vi "Radau5_Initialization of Implicit RK Data.vi"(3 "Simulation Data":T5 {"Absolute tolerance" format="%.1e"; "Relative tolerance" format="%.1e"; "Output of T" format="%.1e"; "proposed step size" format="%.1e"; "min step size" format="%.1e"; "max step size" format="%.1e"; "final time" format="%.1e"; "step size" format="%.1e"; "initial time" format="%.1e"}) -> (1 "Implicit RK Data":T1)   [LabVIEW 2020, in "NI_DAE.lvlib"]
uses:
  <vilib>/gmath/NI_DAE.lvlib
  <vilib>/gmath/dae.llb/Radau5_Simulation Data.ctl
  <vilib>/gmath/dae.llb/Radau5_Diag Eval Stage.ctl
  <vilib>/gmath/dae.llb/Radau5_Implicit RK Data.ctl
  <vilib>/gmath/dae.llb/Radau5_RK Status.ctl
  <vilib>/Analysis/Matrix/Datatypes/RealMatrix.ctl
  <vilib>/Analysis/Matrix/Datatypes/ComplexMatrix.ctl
  <vilib>/Analysis/Matrix/Numeric/Conversions/Array To Matrix - CA2.vi
  <vilib>/Analysis/Matrix/Numeric/Conversions/Array To Matrix - RA2.vi
  <vilib>/Analysis/Matrix/NI_Matrix.lvlib
panel:
  in  "Implicit RK Data Type":T1
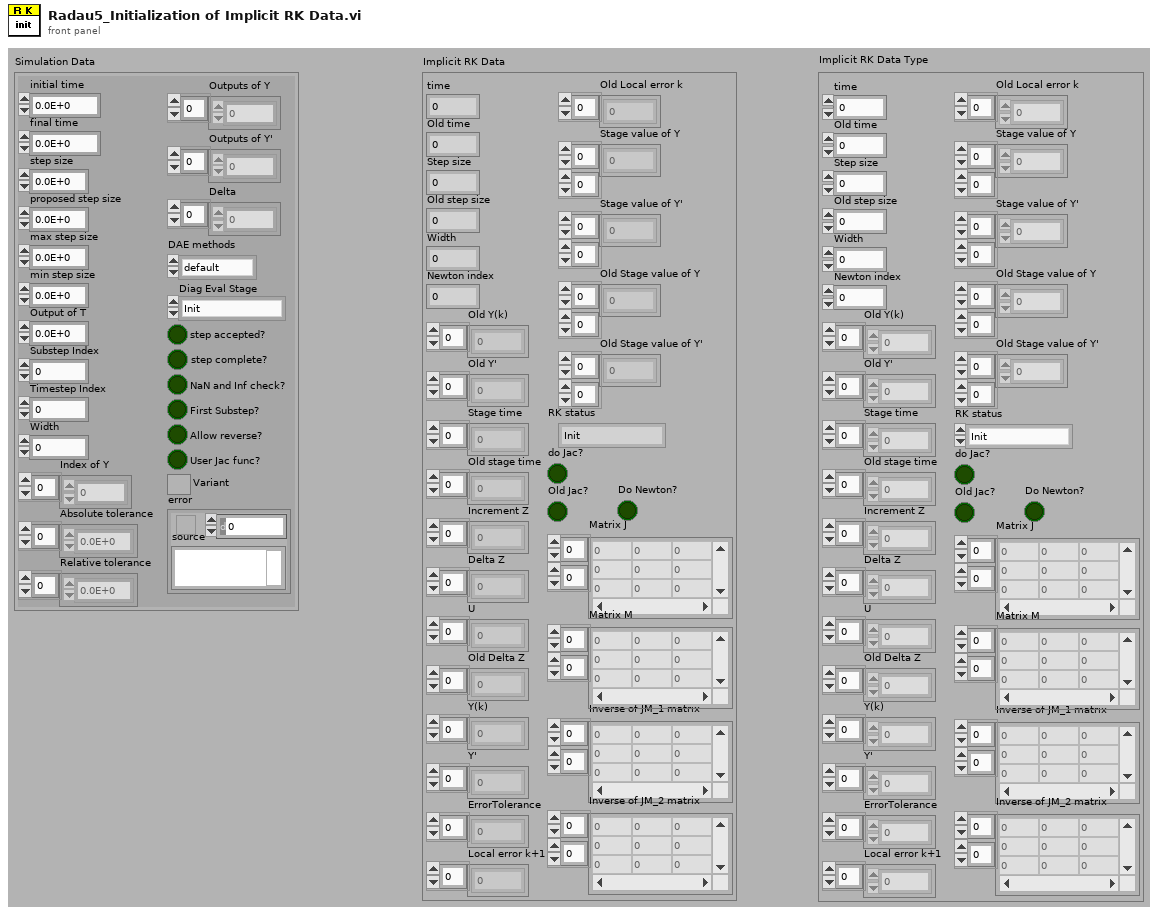
[diagram p1: front panel]
types:
  T1 = typedef "NI_DAE.lvlib/Radau5_Implicit RK Data.ctl" = cluster{"time":dbl, "Old time":dbl, "Step size":dbl, "Old step size":dbl, "Width":i32, "Newton index":i32, "Old Y(k)":dbl[], "Old Y'":dbl[], "Stage time":dbl[], "Old stage time":dbl[], "Increment Z":dbl[], "Delta Z":dbl[], "U":dbl[], "Old Delta Z":dbl[], "Y(k)":dbl[], "Y'":dbl[], "ErrorTolerance":dbl[], "Local error k+1":dbl[], "Old Local error k":dbl[], "Stage value of Y":dbl[][], "Stage value of Y'":dbl[][], "Old Stage value of Y":dbl[][], "Old Stage value of Y'":dbl[][], "RK status":T2, "do Jac?":bool, "Old Jac?":bool, "Do Newton?":bool, "Matrix J":T3, "Matrix M":T3, "Inverse of JM_1 matrix ":T3, "Inverse of JM_2 matrix":T4}
  T2 = typedef "NI_DAE.lvlib/Radau5_RK Status.ctl" = enum16{"Init", "Predict", "Jacobian", "Newton", "error eval y y'", "error eval calc", "next step updata", "reset RK"}
  T3 = typedef "NI_Matrix.lvlib/RealMatrix.ctl" = dbl[][]
  T4 = typedef "NI_Matrix.lvlib/ComplexMatrix.ctl" = cdb[][]
  T5 = typedef "NI_DAE.lvlib/Radau5_Simulation Data.ctl" = cluster{"initial time":dbl, "final time":dbl, "step size":dbl, "proposed step size":dbl, "max step size":dbl, "min step size":dbl, "Output of T":dbl, "Substep Index":i32, "Timestep Index":i32, "Width":i32, "Absolute tolerance":dbl[], "Relative tolerance":dbl[], "Outputs of Y":dbl[], "Outputs of Y'":dbl[], "Delta":dbl[], "DAE methods":enum16{"default", "Radau IIA"}, "Diag Eval Stage":T6, "step accepted?":bool, "step complete?":bool, "NaN and Inf check?":bool, "First Substep?":bool, "Allow reverse?":bool, "error":errorcluster, "User Jac func?":bool, "Variant":variant, "Index of Y":i8[]}
  T6 = typedef "NI_DAE.lvlib/Radau5_Diag Eval Stage.ctl" = enum16{"Init", "Running", "Final", "End"}
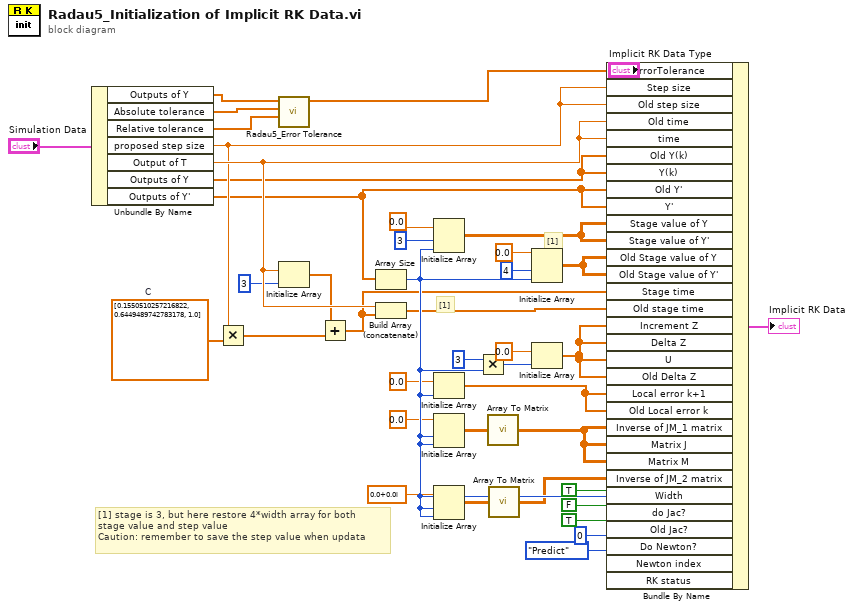
[diagram p0: block diagram]
diagram:
  w3 = dbl[] [0.1550510257216822, 0.6449489742783178, 1.0]  # C
  # "[1]"
  # "[1] stage is 3, but here restore 4*width array for both\nstage value and step value\nCaution: remember to save the step value when updata"
  # "[1]"
  n1 = Unbundle By Name("Simulation Data") -> ("Outputs of Y"=w36:dbl[], "Absolute tolerance"=w30:dbl[], "Relative tolerance"=w31:dbl[], "proposed step size"=w40:dbl, "Output of T"=w41:dbl, "Outputs of Y"=w37:dbl[], "Outputs of Y'"=w34:dbl[])
  n2 = Multiply(x=w40, y=w3) -> (x*y=w21:dbl[])
  n3 = call <vilib>:"Radau5_Error Tolerance.vi"("Relative Tolerance"=w31, "Absolute Tolerance"=w30, "Y in"=w36) -> ("Error tolerance"=w32:dbl[])  [unwired: 8 in]
  n4 = Initialize Array(w41, 3 ("dimension size")) -> (w20:dbl[])
  n5 = Add(x=w20, y=w21) -> (x+y=w25:dbl[])
  n6 = Array Size(array=w34) -> (size(s)=w38:i32)
  n7 = Build Array (concatenate)(w41, w25) -> (w26:dbl[])
  n8 = Initialize Array(0.0, 3 ("dimension size"), w38) -> (w7:dbl[][])
  n9 = Initialize Array(0.0, w38) -> (w29:dbl[])
  n10 = Initialize Array(0.0, w38, w38) -> (w13:dbl[][])
  n11 = Initialize Array(cdb 0.0+0.0i, w38, w38) -> (w14:cdb[][])
  n12 = Multiply(x=3 ("y"), y=w38) -> (x*y=w9:i32)
  n13 = call-poly <vilib>:"Array To Matrix.vi"("Real 2D Array"=w13) -> ("Real Matrix"=w33:T3)
  n14 = call-poly <vilib>:"Array To Matrix.vi"("Complex 2D Array"=w14) -> ("Complex Matrix"=w15:T4)
  n15 = Initialize Array(0.0 ("element"), 4 ("dimension size"), w38) -> (w24:dbl[][])
  n16 = Initialize Array(0.0, w9) -> (w10:dbl[])
  n17 = Bundle By Name(cluster="Implicit RK Data Type", "ErrorTolerance"=w32, "Step size"=w40, "Old step size"=w40, "Old time"=w41, "time"=w41, "Old Y(k)"=w37, "Y(k)"=w37, "Old Y'"=w34, "Y'"=w34, "Stage value of Y"=w7, "Stage value of Y'"=w7, "Old Stage value of Y"=w24, "Old Stage value of Y'"=w24, "Stage time"=w25, "Old stage time"=w26, "Increment Z"=w10, "Delta Z"=w10, "U"=w10, "Old Delta Z"=w10, "Local error k+1"=w29, "Old Local error k"=w29, "Inverse of JM_1 matrix"=w33, "Matrix J"=w33, "Matrix M"=w33, "Inverse of JM_2 matrix"=w15, "Width"=w38, "do Jac?"=TRUE, "Old Jac?"=FALSE, "Do Newton?"=TRUE, "Newton index"=0, "RK status"=Radau5_RK_Status."Predict") -> (→"Implicit RK Data":T1)
